vi "SetUp.vi"(8 "error in (no error)":errorcluster, 11 "Prueba07 in":refnum<class "Prueba07.lvclass">) -> (0 "error out":errorcluster, 3 "Prueba07 out":refnum<class "Prueba07.lvclass">)   [LabVIEW 2019, in "Prueba07.lvclass"]
uses:
  Prueba07.lvclass
  Prueba07.lvclass/Prueba07.ctl
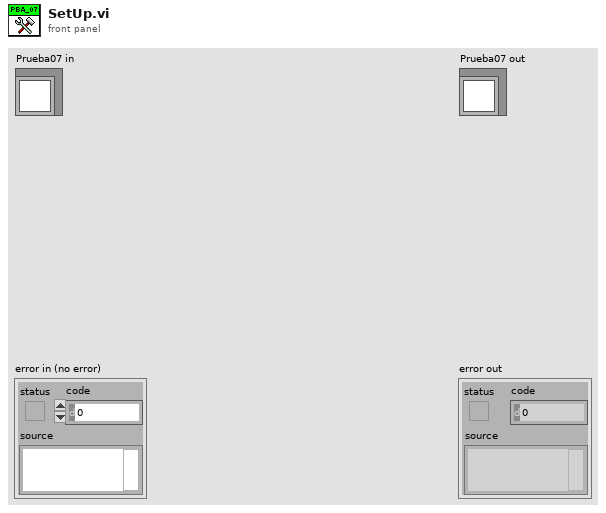
[diagram p1: front panel]
types:
  T1 = typedef "Prueba07.lvclass/BD.ctl" = cluster{"niv_presion_son_ref":dbl, "Incertidumbre":string, "Tol +":string, "Tol -":string, "rangos":string[][], "frecuencia_ref":dbl}
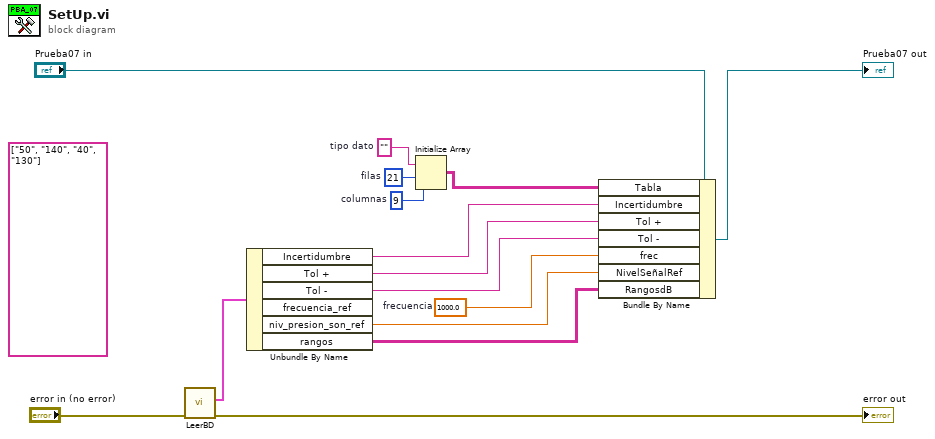
[diagram p0: block diagram]
diagram:
  (unwired) string[][] [["50", "140"], ["40", "130"]]
  w14 = 1000.0  # frecuencia
  w12 = 9  # columnas
  w11 = 21  # filas
  w13 = ""  # tipo dato
  n1 = call "LeerBD.vi"("error in (no error)"="error in (no error)") -> ("error out"=→"error out":errorcluster, "BD"=w6:T1)  [unwired: 8 in, 1 out]
  n2 = Unbundle By Name(w6) -> ("Incertidumbre"=w5:string, "Tol +"=w4:string, "Tol -"=w3:string, "niv_presion_son_ref"=w2:dbl, "rangos"=w1:string[][])  [unwired: 1 out]
  n3 = Initialize Array(w13, w11, w12) -> (w8:string[][])
  n4 = Bundle By Name(cluster="Prueba07 in", "Tabla"=w8, "Incertidumbre"=w5, "Tol +"=w4, "Tol -"=w3, "frec"=w14, "NivelSeñalRef"=w2, "RangosdB"=w1) -> (→"Prueba07 out":refnum<class "Prueba07.lvclass">)
